vi "Launch Nested Actors.vi"(8 "error in (no error)":errorcluster, 11 "Elevator Controller in":refnum<class "Elevator Controller.lvclass">) -> (0 "error out":errorcluster, 3 "Elevator Controller out":refnum<class "Elevator Controller.lvclass">)   [LabVIEW 2019, in "Elevator Controller.lvlib" / "Elevator Controller.lvclass"]
uses:
  Elevator Controller.lvclass
  C:/Program Files (x86)/National Instruments/LabVIEW 2019/vi.lib/ActorFramework/Actor/Actor.lvclass
  Sim User Console Actor/Elevator Controller/Sim User Console Actor.lvclass
  Sim Display Console Actor/Elevator Controller/Sim Display Console Actor.lvclass
  Sim Sensor Interface Actor/Elevator Controller/Sim Sensor Interface Actor.lvclass
  Configuration Database Actor/Configuration Database Actor/Configuration Database Actor.lvclass
  Elevator Controller.lvclass/Elevator Controller.ctl
  <vilib>/ActorFramework/Actor/Actor.lvclass
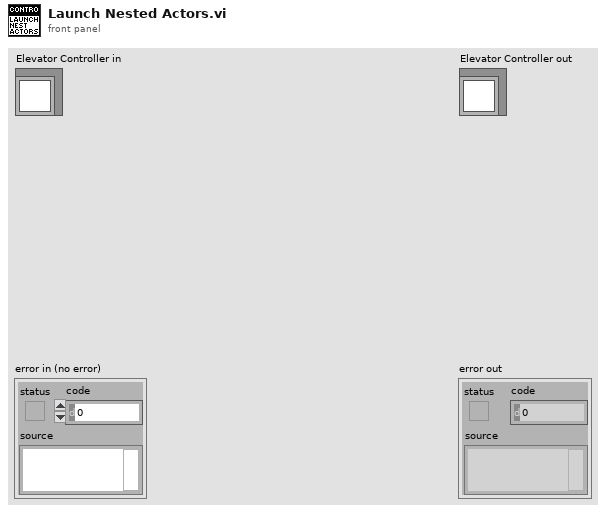
[diagram p1: front panel]
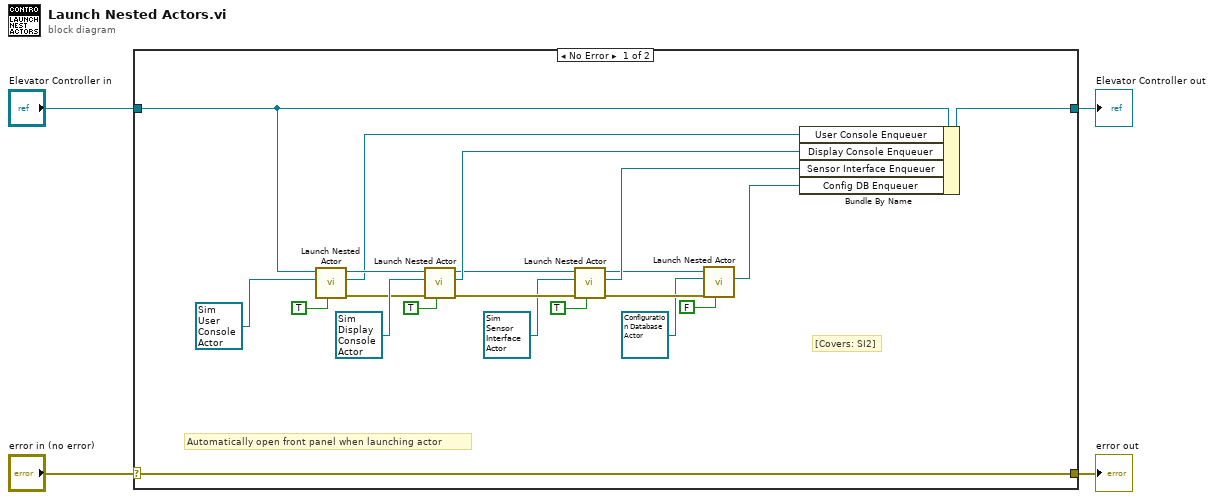
[diagram p0: block diagram]
diagram:
  n1 = case shown="No Error" "error in (no error)" {
    selector: "error in (no error)" -> [w25 w27]
    tunnel: [w25 w27] -> w3
    tunnel: [w20 w26] -> w1
    tunnel: "Elevator Controller in" -> [w21 w26]
    frame No Error {
      # "[Covers: SI2]"
      # "Automatically open front panel when launching actor"
      n2 = call <vilib>:"Launch Nested Actor.vi"("Open Actor Core front panel? (F)"=TRUE, "Nested Actor"=refnum<class "Sim User Console Actor.lvclass"> refnum ("Sim User Console Actor.lvlib:Sim User Console Actor.lvclass"), "Caller Actor in"=w21) -> ("error out"=w11:errorcluster, "Nested Actor's Enqueuer"=w19:refnum<class "Message Enqueuer.lvclass">, "Caller Actor out"=w22:refnum<class "Elevator Controller.lvclass">)  [unwired: 6 in]
      n3 = call <vilib>:"Launch Nested Actor.vi"("Open Actor Core front panel? (F)"=TRUE, "error in (no error)"=w11, "Nested Actor"=refnum<class "Sim Display Console Actor.lvclass"> refnum ("Sim Display Console Actor.lvlib:Sim Display Console Actor.lvclass"), "Caller Actor in"=w22) -> ("error out"=w14:errorcluster, "Nested Actor's Enqueuer"=w16:refnum<class "Message Enqueuer.lvclass">, "Caller Actor out"=w15:refnum<class "Elevator Controller.lvclass">)  [unwired: 5 in]
      n4 = call <vilib>:"Launch Nested Actor.vi"("Open Actor Core front panel? (F)"=TRUE, "error in (no error)"=w14, "Nested Actor"=refnum<class "Sim Sensor Interface Actor.lvclass"> refnum ("Sim Sensor Interface Actor.lvlib:Sim Sensor Interface Actor.lvclass"), "Caller Actor in"=w15) -> ("error out"=w8:errorcluster, "Nested Actor's Enqueuer"=w10:refnum<class "Message Enqueuer.lvclass">, "Caller Actor out"=w9:refnum<class "Elevator Controller.lvclass">)  [unwired: 5 in]
      n5 = call <vilib>:"Launch Nested Actor.vi"("Open Actor Core front panel? (F)"=FALSE, "error in (no error)"=w8, "Nested Actor"=refnum<class "Configuration Database Actor.lvclass"> refnum ("Configuration Database Actor.lvlib:Configuration Database Actor.lvclass"), "Caller Actor in"=w9) -> ("Nested Actor's Enqueuer"=w5:refnum<class "Message Enqueuer.lvclass">)  [unwired: 5 in, 2 out]
      n6 = Bundle By Name(cluster=w21, "User Console Enqueuer"=w19, "Display Console Enqueuer"=w16, "Sensor Interface Enqueuer"=w10, "Config DB Enqueuer"=w5) -> (w20:refnum<class "Elevator Controller.lvclass">)
    }
    frame Error {
    }
  }
  "error out" <- w3
  "Elevator Controller out" <- w1
